vi "Flush Exit.vi"(8 "error in (no error)":errorcluster, 11 "Data":variant) -> (0 "error out":errorcluster)   [LabVIEW 2014, in "RT - Analysis.lvlib"]
doc: "This subVI enqueues the Exit action in to the communications queue along with the input data after flushing the queue."
uses:
  RT - Analysis.lvlib
  Private Controls/Module Data.ctl
  Private Controls/Module Action.ctl
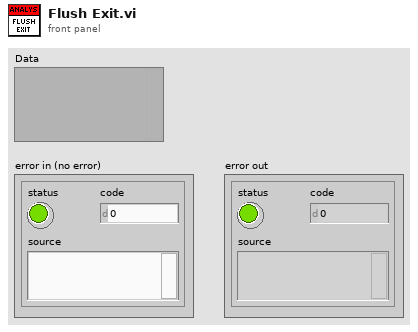
[diagram p1: front panel]
types:
  T1 = typedef "RT - Analysis.lvlib/Module Data.ctl" = cluster{"Data":variant, "Action":T2}
  T2 = typedef "RT - Analysis.lvlib/Module Action.ctl" = enum16{"Check for Data", "Init", "Error", "Exit", "Set APU Setup Info", "Set State", "Set Testing Type", "Set APU Select", "Set Subtests Array", "Set Current Step Index", "Set Confirm Button", "Next SubTest", "Set Fuel Pres Regltr", "Set Bleed-Fuel-ECS Cntrls", "Set ECS Demnd Cluster", "Set APU&ECU Cntrls", "Set Sample Rate", "Threshold ALERT"}
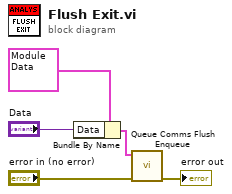
[diagram p0: block diagram]
diagram:
  n1 = Bundle By Name(cluster=T1 {"Data"=variant, "Action"=enum."Exit"} ("element"), "Data"="Data") -> (w1:T1)
  n2 = call "Queue Comms Flush Enqueue.vi"("error in (no error)"="error in (no error)", "element"=w1) -> ("error out"=→"error out":errorcluster)  [unwired: 9 in]
